vi "Main.vi"(8 "error in":errorcluster, 11 "SerialComm in":refnum<class "SerialComm.lvclass">) -> (0 "error out":errorcluster, 3 "SerialComm out":refnum<class "SerialComm.lvclass">)   [LabVIEW 2014, in "SerialComm.lvclass"]
doc: "The Queued Message Handler of a Worker."
uses:
  SerialComm.lvclass
  Initialization Data.ctl
  <vilib>/addons/_Workers/Library/Classes/Worker/Worker.lvclass
  <vilib>/addons/_Workers/Library/Classes/Message/Message.lvclass
  <vilib>/Instr/_visa.llb/VISA Configure Serial Port (Instr).vi
  <vilib>/addons/_Workers/Library/Classes/Message/Enqueue Message to Self v2.vi
  <vilib>/addons/_Workers/Library/Classes/Message/Enqueue Message to Self v2 - Silent Mode.vi
  2a629d3d-49b6-4a3c-83b3-40ed9d97e814.vi
panel:
  out "bytes read":u32
  out "NowTime":timestamp
  in  "ClosePort":bool
  in  "OpenProt":bool
  in  "flow control":u16(ring) items=["None"=0, "XON/XOFF"=1, "RTS/CTS"=2, "DTR/DSR"=4]
  in  "stop bits":u16(ring)=10 items=["1.0"=10, "1.5"=15, "2.0"=20]
  in  "parity":u16(ring) items=["None", "Odd", "Even", "Mark", "Space"]
  in  "data bits":u16=8 min=5 max=8 step=1
  in  "baud rate":u32=9600
  in  "delay before read (ms)":u32=500
  in  "VISA resource name":refnum<visa-resource-name>="COM1"
  out "Response":string
  in  "Command":string="*IDN?\n"
  in  "SerialSend":bool
  out "MsgString":string
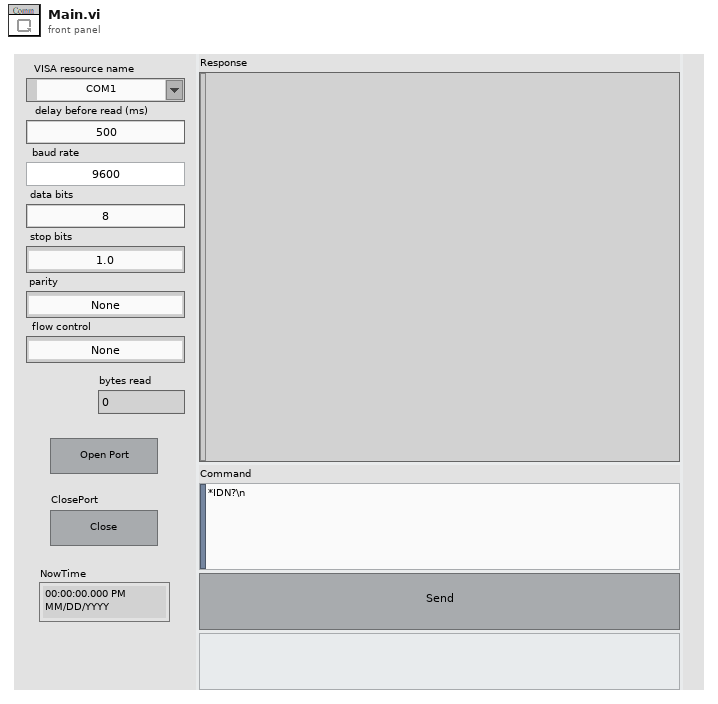
[diagram p1: front panel]
types:
  T1 = typedef "SerialComm.lvclass/Initialization Data.ctl" = cluster{"String":string}
  T2 = typedef "Workers.lvlib/Case Label.ctl" = string
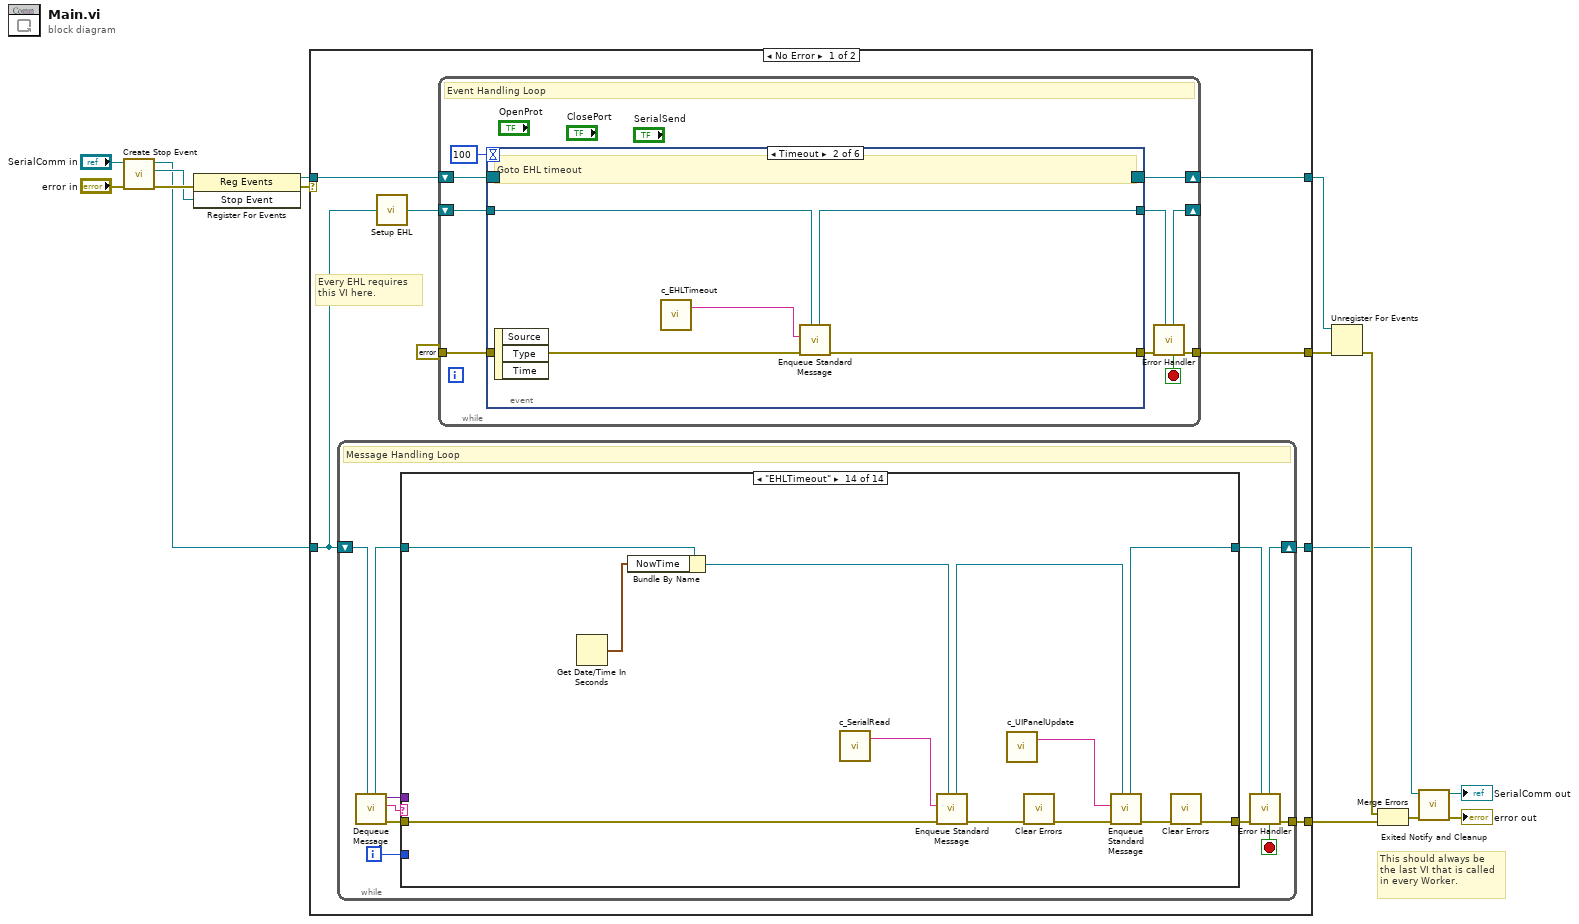
[diagram p0: block diagram]
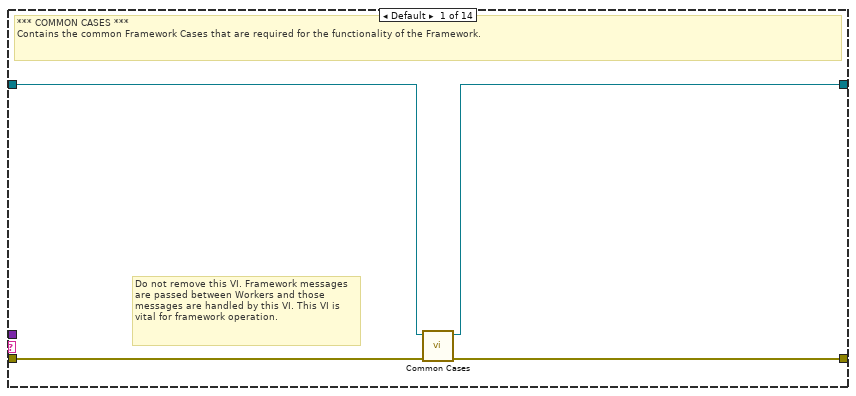
[diagram p2: hidden frame]
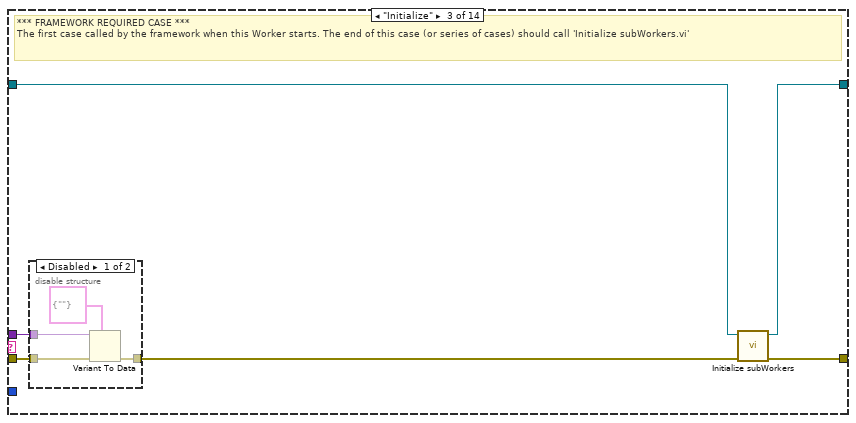
[diagram p4: hidden frame]
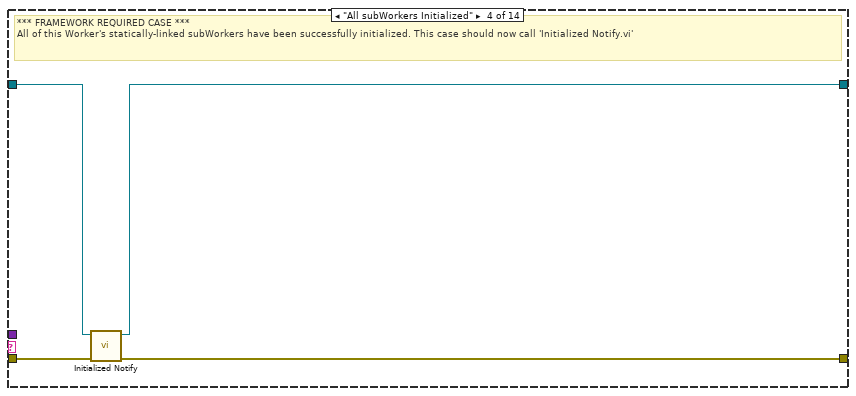
[diagram p6: hidden frame]
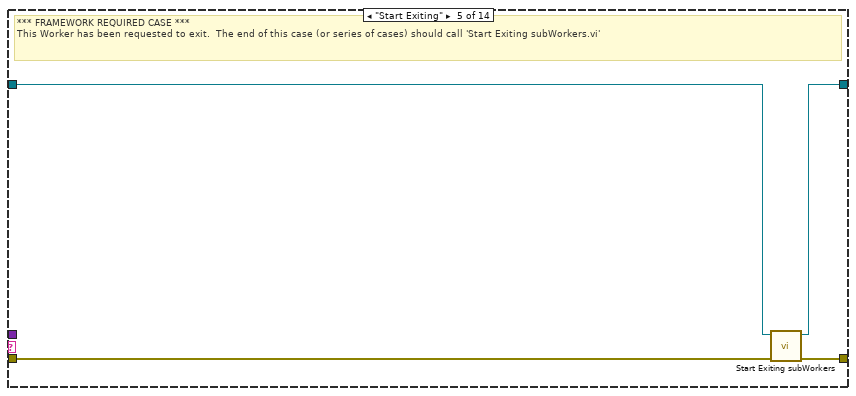
[diagram p7: hidden frame]
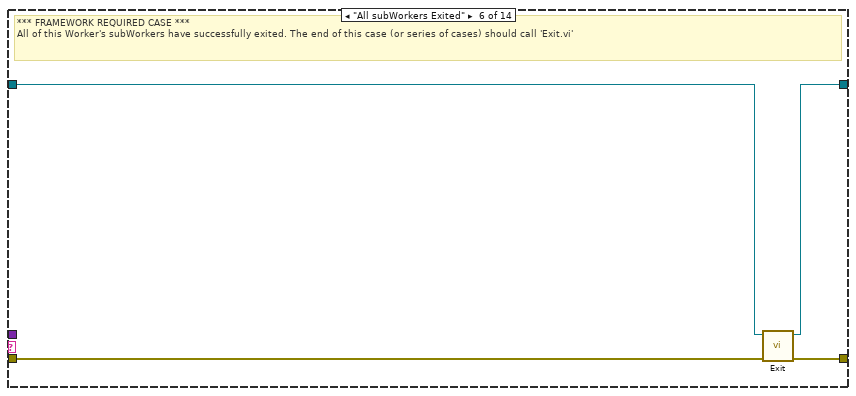
[diagram p8: hidden frame]
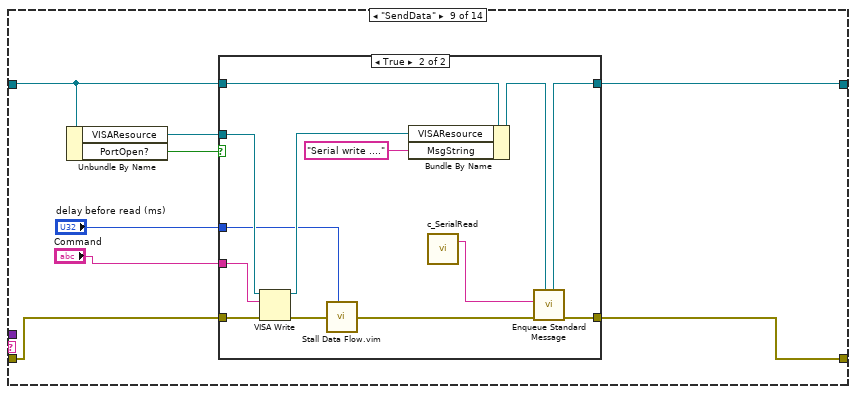
[diagram p11: hidden frame]
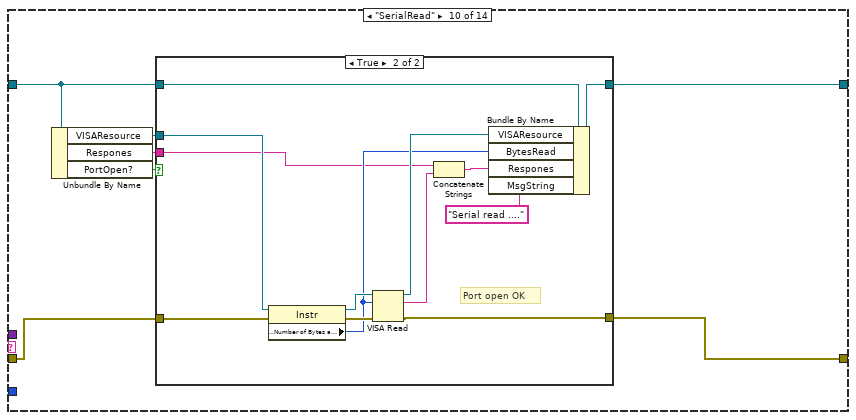
[diagram p13: hidden frame]
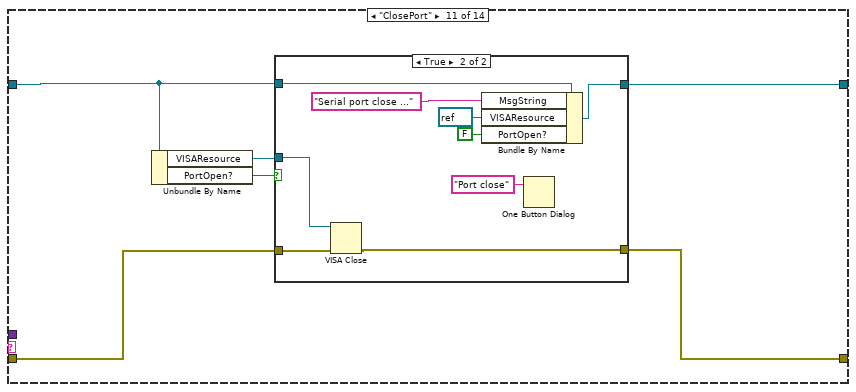
[diagram p15: hidden frame]
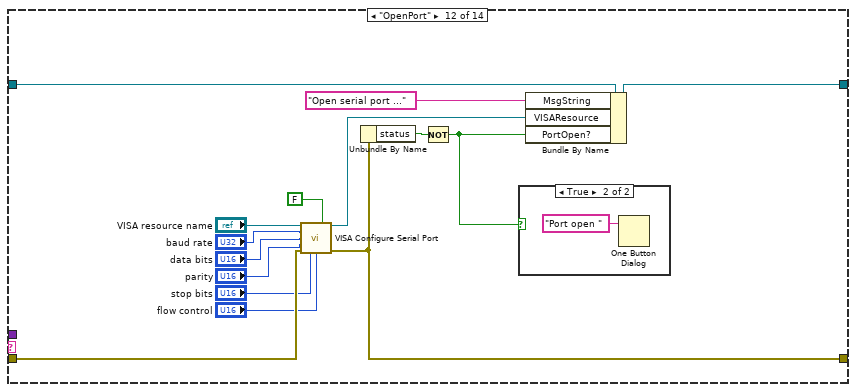
[diagram p17: hidden frame]
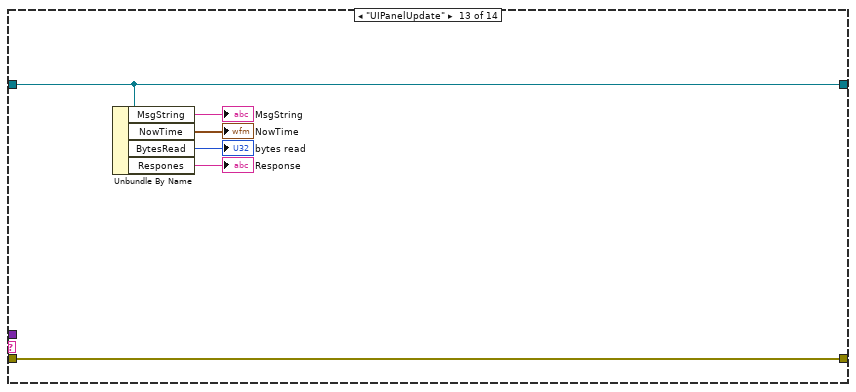
[diagram p19: hidden frame]
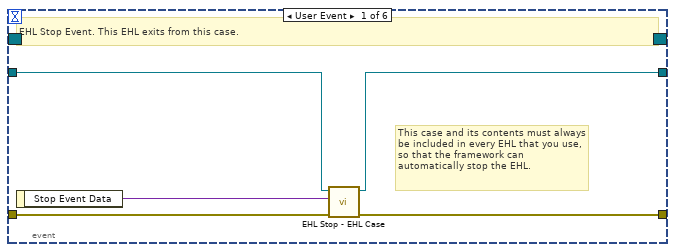
[diagram p20: hidden frame]
diagram:
  # "This should always be the last VI that is called in every Worker."
  n1 = call-dynamic "Create Stop Event.vi"("error in"="error in", "Worker"="SerialComm in") -> ("error out"=w10:errorcluster, "Stop Event"=w7:refnum<user-event>, "Worker out"=w4:refnum<class "SerialComm.lvclass">)  [unwired: 7 in]
  n2 = register-events(error in=w10, w7) -> (reference out=w9:refnum<event-registration>, error out=w1:errorcluster)  [unwired: 1 in]
  n3 = case shown="No Error" w1 {
    tunnel: w4 -> [w18 w205]
    tunnel: [w16 w206] -> w8
    tunnel: w9 -> [w23 w207]
    tunnel: [w20 w208] -> w14
    tunnel: [w22 w207] -> w13
    tunnel: [w17 w204] -> w11
    selector: w1 -> [_ w208]
    frame No Error {
      # "Every EHL requires\nthis VI here."
      n4 = while {
        shift-right: [w32] -> w17
        shift-left: w18 -> [w34]
        tunnel: [w33] -> w16
        i -> [w24]
        stop <- w25 stop-if-true
        # "Message Handling Loop"
        n5 = call-dynamic "Dequeue Message.vi"("Worker"=w34) -> ("error out"=w31:errorcluster, "Case out"=w26:string, "Data out"=w27:variant, "Worker out"=w29:refnum<class "SerialComm.lvclass">)  [unwired: 6 in, 1 out]
        n6 = case "Worker MHL Case Structure (DO NOT CHANGE LABEL NAME)" shown="\"EHLTimeout\"" w26 {
          tunnel: w31 -> [w38 w39 w44 w53 w56 w63 w64 w66 w72 w92 w114 w139 w151 w162]
          tunnel: [w37 w39 w46 w52 w59 w62 w64 w66 w71 w91 w113 w138 w151 w153] -> w30
          tunnel: w29 -> [w36 w40 w43 w55 w57 w61 w65 w67 w73 w94 w116 w144 w150 w163]
          tunnel: [w35 w40 w45 w54 w58 w60 w65 w67 w70 w93 w115 w142 w150 w159] -> w28
          tunnel: w27 -> [_ _ w41 _ _ _ _ _ _ _ _ _ _ _]
          tunnel: w24 -> [_ _ _ _ _ _ _ _ _ _ _ _ _ _]
          frame Default {
            # "Do not remove this VI. Framework messages are passed between Workers and those messages are handled by this VI. This VI is vital for framework operation."
            # "*** COMMON CASES ***\nContains the common Framework Cases that are required for the functionality of the Framework."
            n7 = call-dynamic "Common Cases.vi"("error in"=w38, "Worker in"=w36) -> ("error out"=w37:errorcluster, "Worker out"=w35:refnum<class "SerialComm.lvclass">)  [unwired: 8 in]
          }
          frame "------ FRAMEWORK REQUIRED CASES ------" {
            # "Start of Framework Required Cases"
          }
          frame "Initialize" {
            # "*** FRAMEWORK REQUIRED CASE ***\nThe first case called by the framework when this Worker starts. The end of this case (or series of cases) should call 'Initialize subWorkers.vi'"
            n8 = disable-structure shown="Disabled" {
              disable-tunnel: w44 -> [w50 w51]
              disable-tunnel: [w49 w51] -> w42
              disable-tunnel: w41 -> [w48 _]
              frame Disabled {
                n9 = Variant To Data(error in=w50, type=T1 {"String"=""} ("Initialization Data"), Variant=w48) -> (error out=w49:errorcluster)  [unwired: 1 out]
              }
              frame Enabled {
              }
            }
            n10 = call-dynamic "Initialize subWorkers.vi"("error in"=w42, "Worker"=w43) -> ("error out"=w46:errorcluster, "dup Worker out"=w45:refnum<class "SerialComm.lvclass">)  [unwired: 8 in]
          }
          frame "All subWorkers Initialized" {
            # "*** FRAMEWORK REQUIRED CASE ***\nAll of this Worker's statically-linked subWorkers have been successfully initialized. This case should now call 'Initialized Notify.vi'"
            n11 = call-dynamic "Initialized Notify.vi"("error in"=w53, "Worker"=w55) -> ("error out"=w52:errorcluster, "dup Worker out"=w54:refnum<class "SerialComm.lvclass">)  [unwired: 8 in]
          }
          frame "Start Exiting" {
            # "*** FRAMEWORK REQUIRED CASE ***\nThis Worker has been requested to exit.  The end of this case (or series of cases) should call 'Start Exiting subWorkers.vi'"
            n12 = call-dynamic "Start Exiting subWorkers.vi"("error_in"=w56, "Worker"=w57) -> ("error out"=w59:errorcluster, "dup Worker out"=w58:refnum<class "SerialComm.lvclass">)  [unwired: 8 in]
          }
          frame "All subWorkers Exited" {
            # "*** FRAMEWORK REQUIRED CASE ***\nAll of this Worker's subWorkers have successfully exited. The end of this case (or series of cases) should call 'Exit.vi'"
            n13 = call-dynamic "Exit.vi"("error_in"=w63, "Worker"=w61) -> ("error out"=w62:errorcluster, "dup Worker out"=w60:refnum<class "SerialComm.lvclass">)  [unwired: 8 in]
          }
          frame "-----------------------------------------------" {
            # "End of Framework Required Cases"
          }
          frame "empty" {
          }
          frame "SendData" {
            n14 = Unbundle By Name(w73) -> ("VISAResource"=w75:refnum<visa-resource-name>, "PortOpen?"=w74:bool)
            n15 = case shown="True" w74 {
              tunnel: w73 -> [w77 w90]
              tunnel: w75 -> [_ w88]
              tunnel: w72 -> [w76 w86]
              tunnel: [w77 w83] -> w70
              tunnel: [w76 w80] -> w71
              tunnel: "Command" -> [_ w79]
              tunnel: "delay before read (ms)" -> [_ w78]
              frame False {
                # "Port not open"
              }
              frame True {
                n16 = VISA Write(VISA resource name=w88, write buffer=w79, error in (no error)=w86) -> (VISA resource name out=w87:refnum<visa-resource-name>, error out=w85:errorcluster)  [unwired: 1 out]
                n17 = call "Stall Data Flow.vim"("value in"=w85, "milliseconds to wait"=w78) -> ("value out"=w81:errorcluster)  [unwired: 1 out]
                n18 = Bundle By Name(cluster=w90, "VISAResource"=w87, "MsgString"="Serial write ....") -> (w84:refnum<class "SerialComm.lvclass">)
                n19 = call "c_SerialRead.vi"() -> ("Case Label"=w82:T2)  [unwired: 1 in]
                n20 = call-poly <vilib>:"Enqueue Standard Message.vi"("Worker"=w84, "error in"=w81, "Case Label"=w82) -> ("error out"=w80:errorcluster, "dup Worker out"=w83:refnum<class "SerialComm.lvclass">)  [unwired: 7 in]
              }
            }
          }
          frame "SerialRead" {
            n21 = Unbundle By Name(w94) -> ("VISAResource"=w97:refnum<visa-resource-name>, "Respones"=w96:string, "PortOpen?"=w95:bool)
            n22 = case shown="True" w95 {
              tunnel: w94 -> [w99 w110]
              tunnel: w97 -> [_ w109]
              tunnel: w92 -> [w98 w108]
              tunnel: [w99 w107] -> w93
              tunnel: w96 -> [_ w102]
              tunnel: [w98 w100] -> w91
              frame False {
                # "Port not open"
              }
              frame True {
                # "Port open OK"
                n23 = property class="Instr"(reference=w109, error in=w108) -> (reference out=w111:refnum<visa-resource-name>, error out=w112:errorcluster, "Serial Settings:Number of Bytes at Serial Port"=w105:u32)
                n24 = VISA Read(VISA resource name=w111, byte count=w105, error in (no error)=w112) -> (VISA resource name out=w106:refnum<visa-resource-name>, read buffer=w104:string, error out=w100:errorcluster)  [unwired: 1 out]
                n25 = Concatenate Strings(w102, w104) -> (w103:string)
                n26 = Bundle By Name(cluster=w110, "VISAResource"=w106, "BytesRead"=w105, "Respones"=w103, "MsgString"="Serial read ....") -> (w107:refnum<class "SerialComm.lvclass">)
              }
            }
          }
          frame "ClosePort" {
            n27 = Unbundle By Name(w116) -> ("VISAResource"=w117:refnum<visa-resource-name>, "PortOpen?"=w118:bool)
            n28 = case shown="True" w118 {
              tunnel: [w120 w129] -> w115
              tunnel: w116 -> [w120 w127]
              tunnel: w117 -> [_ w126]
              tunnel: w114 -> [w119 w125]
              tunnel: [w119 w122] -> w113
              frame False {
                # "port not open"
              }
              frame True {
                n29 = VISA Close(VISA resource name=w126, error in (no error)=w125) -> (error out=w122:errorcluster)
                n30 = Bundle By Name(cluster=w127, "MsgString"="Serial port close ..." ("message"), "VISAResource"=refnum<visa-resource-name> refnum, "PortOpen?"=FALSE) -> (w129:refnum<class "SerialComm.lvclass">)
                n31 = One Button Dialog(message="Port close") -> ()  [unwired: 1 in, 1 out]
              }
            }
          }
          frame "OpenPort" {
            n32 = call-poly "VISA Configure Serial Port"("VISA resource name"="VISA resource name", "Enable Termination\nChar (T)"=FALSE ("Enable Termination\nChar (T)"), "baud rate (9600)"="baud rate", "data bits (8)"="data bits", "parity (0:none)"="parity", "error in (no error)"=w139, "stop bits (10: 1 bit)"="stop bits", "flow control (0:none)"="flow control") -> ("VISA resource name out"=w140:refnum<visa-resource-name>, "error out"=w138:errorcluster)  [unwired: 1 in, 5 out]
            n33 = Unbundle By Name(w138) -> ("status"=w143:bool)
            n34 = Not(x=w143) -> (.not. x?=w130:bool)
            n35 = case shown="True" w130 {
              frame False {
              }
              frame True {
                n36 = One Button Dialog(message="Port open ") -> ()  [unwired: 1 in, 1 out]
              }
            }
            n37 = Bundle By Name(cluster=w144, "MsgString"="Open serial port ..." ("message"), "VISAResource"=w140, "PortOpen?"=w130) -> (w142:refnum<class "SerialComm.lvclass">)
          }
          frame "UIPanelUpdate" {
            n38 = Unbundle By Name(w150) -> ("MsgString"=→"MsgString":string, "NowTime"=→"NowTime":timestamp, "BytesRead"=→"bytes read":u32, "Respones"=→"Response":string)
          }
          frame "EHLTimeout" {
            n39 = Get Date/Time In Seconds() -> (seconds since 1Jan1904=w161:timestamp)
            n40 = Bundle By Name(cluster=w163, "NowTime"=w161) -> (w155:refnum<class "SerialComm.lvclass">)
            n41 = call "c_SerialRead.vi"() -> ("Case Label"=w154:T2)  [unwired: 1 in]
            n42 = call-poly <vilib>:"Enqueue Standard Message.vi"("Worker"=w155, "error in"=w162, "Case Label"=w154) -> ("error out"=w157:errorcluster, "dup Worker out"=w156:refnum<class "SerialComm.lvclass">)  [unwired: 7 in]
            n43 = call "c_UIPanelUpdate.vi"() -> ("Case Label"=w158:T2)  [unwired: 1 in]
            n44 = call <vilib>:"Clear Errors.vi"("error in (no error)"=w157) -> ("error out"=w152:errorcluster)  [unwired: 5 in, 1 out]
            n45 = call-poly <vilib>:"Enqueue Standard Message.vi"("Worker"=w156, "error in"=w152, "Case Label"=w158) -> ("error out"=w160:errorcluster, "dup Worker out"=w159:refnum<class "SerialComm.lvclass">)  [unwired: 7 in]
            n46 = call <vilib>:"Clear Errors.vi"("error in (no error)"=w160) -> ("error out"=w153:errorcluster)  [unwired: 5 in, 1 out]
          }
        }
        n47 = call-dynamic "Error Handler.vi"("Worker"=w28, "error_in"=w30) -> ("error out"=w33:errorcluster, "Stop Loop"=w25:bool, "Worker out"=w32:refnum<class "SerialComm.lvclass">)  [unwired: 7 in]
      }
      n48 = call-dynamic "Setup EHL.vi"("Worker"=w18) -> ("Worker out"=w19:refnum<class "SerialComm.lvclass">)  [unwired: 14 in]
      n49 = while "Event Handling Loop" {
        shift-right: [w173] -> w22
        shift-left: w23 -> [w172]
        tunnel: [w168] -> w20
        tunnel: errorcluster {"status"=FALSE, "code"=0, "source"=""} ("error constant") -> [w170]
        shift-right: [w166] -> _
        shift-left: w19 -> [w171]
        stop <- w165 stop-if-true
        # "Event Handling Loop"
        n50 = event shown="[1] Timeout" {
          selector: w172 -> [_ _ _ _ _ _]
          dyn-events: [_ _ _ _ _ _] -> w173
          timeout: 100 -> [_ _ _ _ _ _]
          tunnel: [w177 w182 w187 w192 w197 w202] -> w169
          tunnel: w170 -> [w178 w183 w188 w193 w198 w201]
          tunnel: w171 -> [w176 w181 w186 w191 w196 w200]
          tunnel: [w175 w180 w185 w190 w195 w199] -> w167
          event User Event {
            # "This case and its contents must always be included in every EHL that you use, so that the framework can automatically stop the EHL."
            # "EHL Stop Event. This EHL exits from this case."
            n51 = event-data() -> ("Stop Event Data"=w174:variant)  [unwired: 1 in]
            n52 = call <vilib>:"EHL Stop - EHL Case.vi"("error in"=w178, "Stop Event Data"=w174, "Worker"=w176) -> ("error out"=w177:errorcluster, "Worker out"=w175:refnum<class "SerialComm.lvclass">)  [unwired: 7 in]
          }
          event Timeout {
            # "Goto EHL timeout"
            n53 = event-data() -> ()  [unwired: 1 in, 3 out]
            n54 = call "c_EHLTimeout.vi"() -> ("Case Label"=w179:T2)  [unwired: 1 in]
            n55 = call-poly <vilib>:"Enqueue Standard Message.vi"("Worker"=w181, "error in"=w183, "Case Label"=w179) -> ("error out"=w182:errorcluster, "dup Worker out"=w180:refnum<class "SerialComm.lvclass">)  [unwired: 7 in]
          }
          event "OpenProt": Value Change {
            n56 = event-data() -> ()  [unwired: 1 in, 4 out]
            n57 = call "c_OpenPort.vi"() -> ("Case Label"=w184:T2)  [unwired: 1 in]
            n58 = call-poly <vilib>:"Enqueue Standard Message.vi"("Worker"=w186, "error in"=w188, "Case Label"=w184) -> ("error out"=w187:errorcluster, "dup Worker out"=w185:refnum<class "SerialComm.lvclass">)  [unwired: 7 in]
          }
          event "ClosePort": Value Change {
            n59 = event-data() -> ()  [unwired: 1 in, 4 out]
            n60 = call "c_ClosePort.vi"() -> ("Case Label"=w189:T2)  [unwired: 1 in]
            n61 = call-poly <vilib>:"Enqueue Standard Message.vi"("Worker"=w191, "error in"=w193, "Case Label"=w189) -> ("error out"=w192:errorcluster, "dup Worker out"=w190:refnum<class "SerialComm.lvclass">)  [unwired: 7 in]
          }
          event "SerialSend": Value Change {
            n62 = event-data() -> ()  [unwired: 1 in, 4 out]
            n63 = call "c_SendData.vi"() -> ("Case Label"=w194:T2)  [unwired: 1 in]
            n64 = call-poly <vilib>:"Enqueue Standard Message.vi"("Worker"=w196, "error in"=w198, "Case Label"=w194) -> ("error out"=w197:errorcluster, "dup Worker out"=w195:refnum<class "SerialComm.lvclass">)  [unwired: 7 in]
          }
          event Panel Close? {
            # "Use this VI when you want to exit this Worker. This VI will call the Start Exiting case of this Worker. This is the recommened way to exit your Worker."
            # "Calls the Start Exiting case of this Worker. This will start the exiting sequence of this Worker."
            n65 = event-data() -> ()  [unwired: 1 in, 1 out]
            n66 = call-dynamic "Start Exiting Worker.vi"("error in"=w201, "Worker"=w200) -> ("error out"=w202:errorcluster, "dup Worker out"=w199:refnum<class "SerialComm.lvclass">)  [unwired: 8 in]
            n67 = event-data("Discard?"=TRUE) -> ()  [unwired: 1 in, 1 out]
          }
        }
        n68 = call-dynamic "Error Handler.vi"("Worker"=w167, "error_in"=w169) -> ("error out"=w168:errorcluster, "Stop Loop"=w165:bool, "Worker out"=w166:refnum<class "SerialComm.lvclass">)  [unwired: 7 in]
      }
    }
    frame Error {
      n69 = call-dynamic "Error Handler.vi"("Worker"=w205, "error_in"=w208) -> ("error out"=w206:errorcluster, "Worker out"=w204:refnum<class "SerialComm.lvclass">)  [unwired: 7 in, 1 out]
    }
  }
  n70 = Unregister For Events(event registration refnum=w13, error in=w14) -> (error out=w15:errorcluster)
  n71 = Merge Errors(w15, w8) -> (w12:errorcluster)
  n72 = call-dynamic "Exited Notify and Cleanup.vi"("error_in"=w12, "Worker"=w11) -> ("error out"=→"error out":errorcluster, "dup Worker out"=→"SerialComm out":refnum<class "SerialComm.lvclass">)  [unwired: 8 in]
